vi "Create Starting Points.vi"(11 "Grid":string[][](array[string])) -> (3 "Starting Points":T1(array[cluster]))   [LabVIEW 2021]
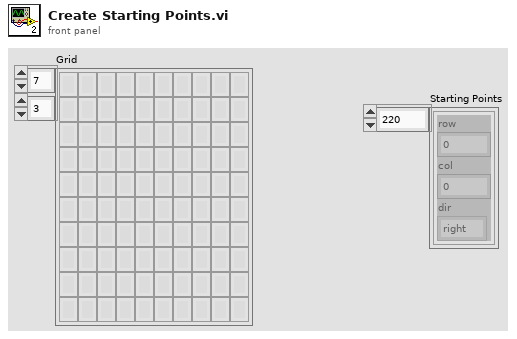
[diagram p1: front panel]
types:
  T1 = cluster{"row":i32, "col":i32, "dir":enum16{"right", "left", "up", "down"}}[]
  T2 = cluster{"row":i32, "col":i32, "dir":enum16{"right", "left", "up", "down"}}
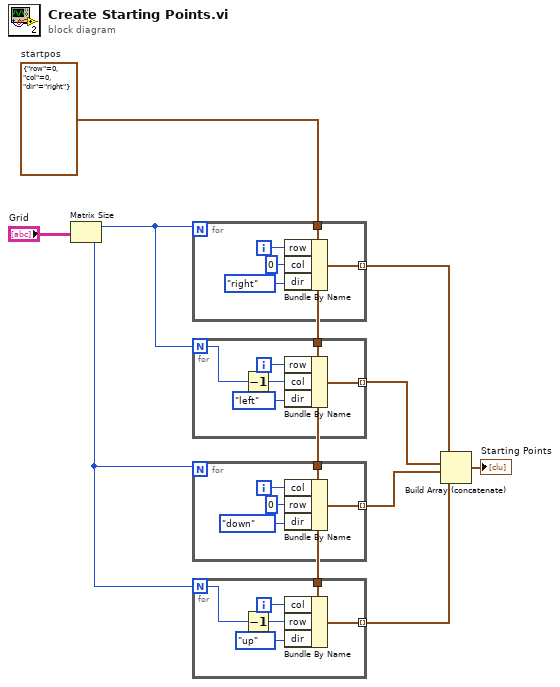
[diagram p0: block diagram]
diagram:
  w7 = T2 {"row"=0, "col"=0, "dir"=enum."right"}  # startpos
  n1 = Matrix Size(0:"Grid") -> (1:w8:i32, 2:w6:i32)
  n2 = for {
    N: w8 -> [_]
    tunnel: w7 -> [w14]
    tunnel: [w10] -> w2 mode=indexing
    i -> [w13]
    n3 = Bundle By Name(cluster=w14, "row"=w13, "col"=0, "dir"=enum16{"right", "left", "up", "down"}."right") -> (w10:T2)
  }
  n4 = for {
    N: w8 -> [w16]
    tunnel: w7 -> [w20]
    tunnel: [w17] -> w3 mode=indexing
    i -> [w19]
    n5 = Decrement(x=w16) -> (x-1=w15:i32)
    n6 = Bundle By Name(cluster=w20, "row"=w19, "col"=w15, "dir"=enum16{"right", "left", "up", "down"}."left") -> (w17:T2)
  }
  n7 = for {
    N: w6 -> [_]
    tunnel: w7 -> [w25]
    tunnel: [w21] -> w4 mode=indexing
    i -> [w24]
    n8 = Bundle By Name(cluster=w25, "col"=w24, "row"=0 ("col"), "dir"=enum16{"right", "left", "up", "down"}."down") -> (w21:T2)
  }
  n9 = for {
    N: w6 -> [w27]
    tunnel: w7 -> [w31]
    tunnel: [w28] -> w5 mode=indexing
    i -> [w30]
    n10 = Decrement(x=w27) -> (x-1=w26:i32)
    n11 = Bundle By Name(cluster=w31, "col"=w30, "row"=w26, "dir"=enum16{"right", "left", "up", "down"}."up") -> (w28:T2)
  }
  n12 = Build Array (concatenate)(w2, w3, w4, w5) -> (→"Starting Points":T1)
